vi "Sam_OpenVINO_advanced.vi"() -> ()   [LabVIEW 2018]
doc: "Sam_OpenVINO_Advanced: This example showcases advanced segmentation capabilities using the SAM (Segment Anything Model) integrated with OpenVINO for optimized performance. This implementation enables precise and customizable image segmentation, allowing users to:\n\nSelect Regions of Interest (ROI): Define areas of interest to focus on specific parts of the image for segmentation.\nExclude Regions of Non-Interest: Mark areas to exclude from segmentation, providing flexibility to ignore irrelevant regions.\nCustomizable Segmentation Regions: Choose specific segments within the image for detailed analysis or processing.\nThis advanced segmentation functionality is particularly useful for applications such as medical imaging, industrial inspection, and autonomous systems, where detailed and flexible segmentation is critical. OpenVINO ensures efficient real-time inference, making it suitable for large-scale deployment across diverse hardware platforms."
uses:
  vi.lib/VIRobotics/ModelZoo/Segmentation/Segment_Anything_Utils/sam_mode.ctl
  vi.lib/VIRobotics/opencv_yiku/ctls/ColorConversionCodes.ctl
  vi.lib/VIRobotics/ModelZoo/Segmentation/Segment_Anything_OpenVINO/Segment_Anything_OpenVINO.lvclass
  C:/Program Files/National Instruments/LabVIEW 2018/vi.lib/VIRobotics/ModelZoo/Segmentation/Segment_Anything_Utils/Segment_Anything_Utils.lvclass
  vi.lib/VIRobotics/opencv_yiku/Mat/Mat_8U/Mat_8U.lvclass
  C:/Program Files/National Instruments/LabVIEW 2018/vi.lib/VIRobotics/opencv_yiku/Mat/Mat/Mat.lvclass
  vi.lib/VIRobotics/ModelZoo/Segmentation/Segment_Anything_Utils/set_mode.vi
  vi.lib/VIRobotics/opencv_yiku/Mat/Create_Mat_8U.vi
  vi.lib/VIRobotics/ModelZoo/Segmentation/Segment_Anything_Utils/set_point.vi
  vi.lib/VIRobotics/ModelZoo/Segmentation/Segment_Anything_Utils/set_labels.vi
  vi.lib/VIRobotics/opencv_yiku/Mat/Create_Mat_8UC3_Size.vi
  vi.lib/VIRobotics/opencv_yiku/Mat/Mat/Mat_release.vi
  vi.lib/VIRobotics/opencv_yiku/Mat/Mat/Mat.lvclass
  vi.lib/VIRobotics/opencv_yiku/opencv_yiku.lvlib
  vi.lib/VIRobotics/ModelZoo/Segmentation/Segment_Anything_Utils/Segment_Anything_Utils.lvclass
panel:
  in  "point type":T1(ring)=enum."included"
  in  "decodr_config":cluster{"decoder_model":path, "device":string}={"decoder_model"=path "C:/ProgramData/VIRobotics/ModelZoo/Segmentation/sam/sam-b-dec.onnx", "device"="CPU"}
  in  "encoder_config":cluster{"encoder_model":path, "device":string}={"encoder_model"=path "C:/ProgramData/VIRobotics/ModelZoo/Segmentation/sam/sam-b-enc.onnx", "device"="CPU"}
  in  "img":path=path "C:/ProgramData/VIRobotics/ModelZoo/Segmentation/imgs/plant.jpg"
  out "picture":picture
  out "x-y":dbl
  out "mask":picture
  in  "run":bool
  # "Overview: Demonstrates how to use the VIRobotics openvino toolkit to load the ONNX model of sam for Semantic segmentation annotation\nRequirements: Windows.\nInstructions: \n1.Run the VI.\n2.Specify the image that requires segmentation annotation。\n3.Specify the point type.\n4.Click on the target with the mouse on the picture control\n5.Click run"
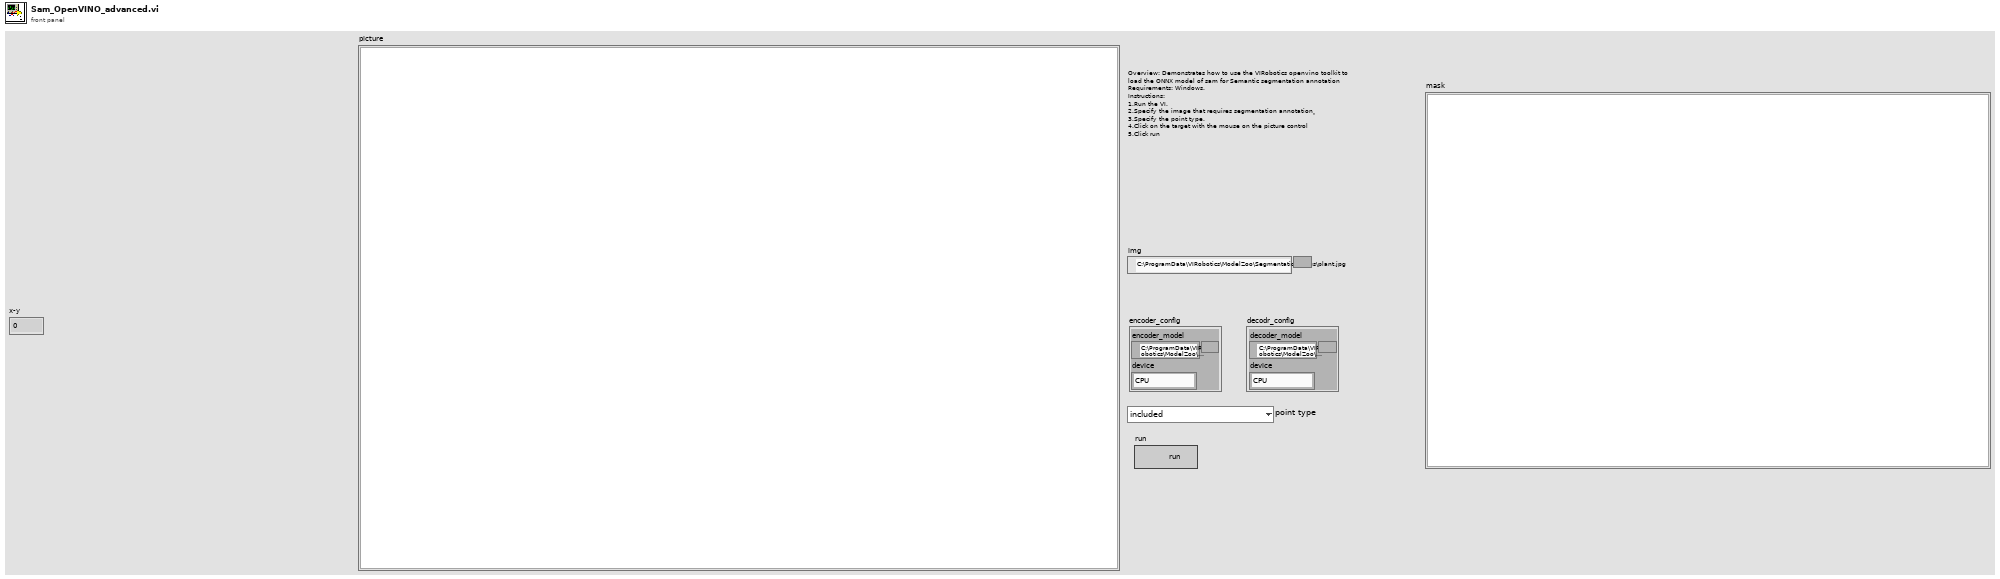
[diagram p1: front panel]
types:
  T1 = enum16{"not included", "included", "top left corner", "bottom right corner"}
  T2 = typedef "Segment_Anything_Utils.lvclass/sam_mode.ctl" = enum16{"points", "box_point", "customize"}
  T3 = typedef "opencv_yiku.lvlib/ColorConversionCodes.ctl" = enum32{"COLOR_BGR2BGRA", "COLOR_BGRA2BGR", "COLOR_BGR2RGBA", "COLOR_RGBA2BGR", "COLOR_BGR2RGB", "COLOR_BGRA2RGBA", "COLOR_BGR2GRAY", "COLOR_RGB2GRAY", "COLOR_GRAY2BGR", "COLOR_GRAY2BGRA", "COLOR_BGRA2GRAY", "COLOR_RGBA2GRAY", "COLOR_BGR2BGR565", "COLOR_RGB2BGR565", "COLOR_BGR5652BGR", "COLOR_BGR5652RGB", "COLOR_BGRA2BGR565", "COLOR_RGBA2BGR565", "COLOR_BGR5652BGRA", "COLOR_BGR5652RGBA", "COLOR_GRAY2BGR565", "COLOR_BGR5652GRAY", "COLOR_BGR2BGR555", "COLOR_RGB2BGR555", "COLOR_BGR5552BGR", "COLOR_BGR5552RGB", "COLOR_BGRA2BGR555", "COLOR_RGBA2BGR555", "COLOR_BGR5552BGRA", "COLOR_BGR5552RGBA", "COLOR_GRAY2BGR555", "COLOR_BGR5552GRAY", "COLOR_BGR2XYZ", "COLOR_RGB2XYZ", "COLOR_XYZ2BGR", "COLOR_XYZ2RGB", "COLOR_BGR2YCrCb", "COLOR_RGB2YCrCb", "COLOR_YCrCb2BGR", "COLOR_YCrCb2RGB", "COLOR_BGR2HSV", "COLOR_RGB2HSV", "42", "43", "COLOR_BGR2Lab", "COLOR_RGB2Lab"}
  T4 = typedef "LVBoundsTypeDef.ctl" = cluster{"Width":u32, "Height":u32}
  T5 = typedef "LVMouseTypeDef.ctl" = cluster{"Mouse Position":cluster{"X":i32, "Y":i32}, "Mouse Modifiers":cluster{"Button Down":bool, "Shift Mod":bool, "Menu Mod":bool, "Option Mod":bool}}
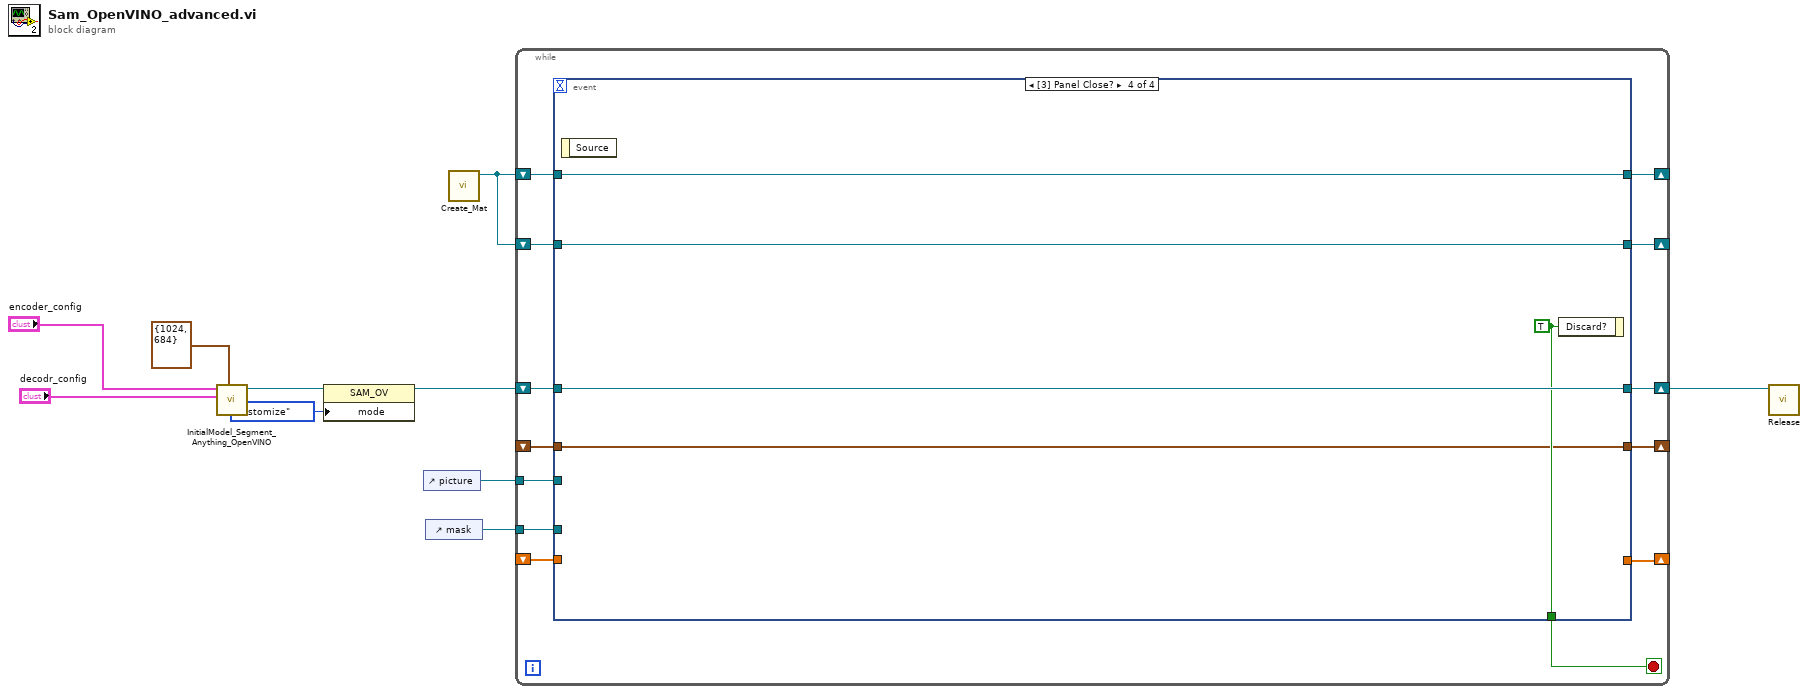
[diagram p0: block diagram]
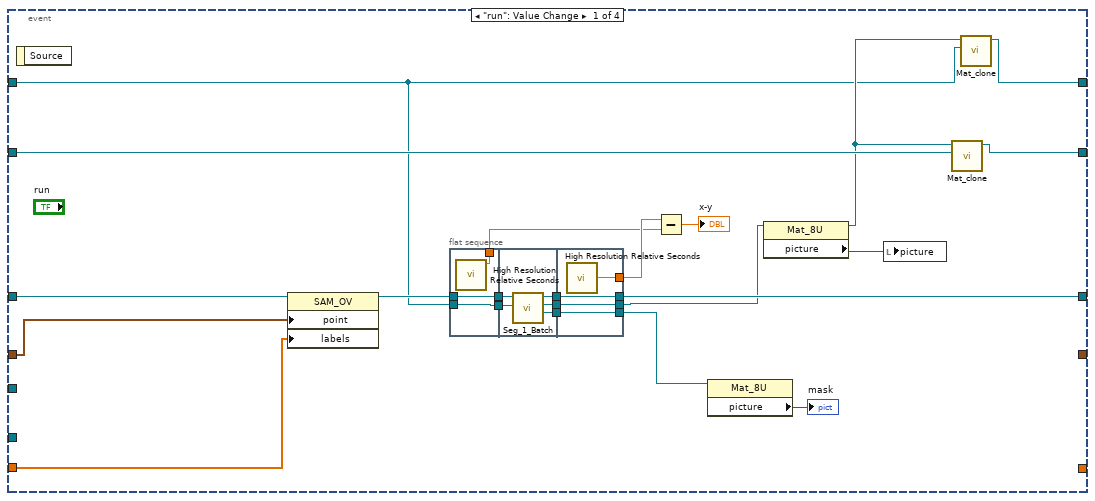
[diagram p2: hidden frame]
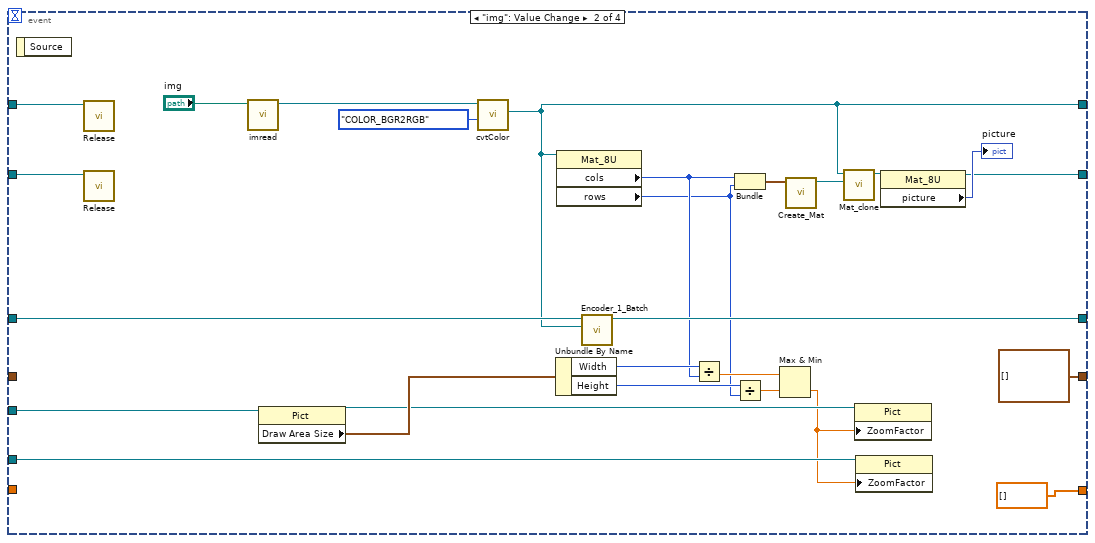
[diagram p3: hidden frame]
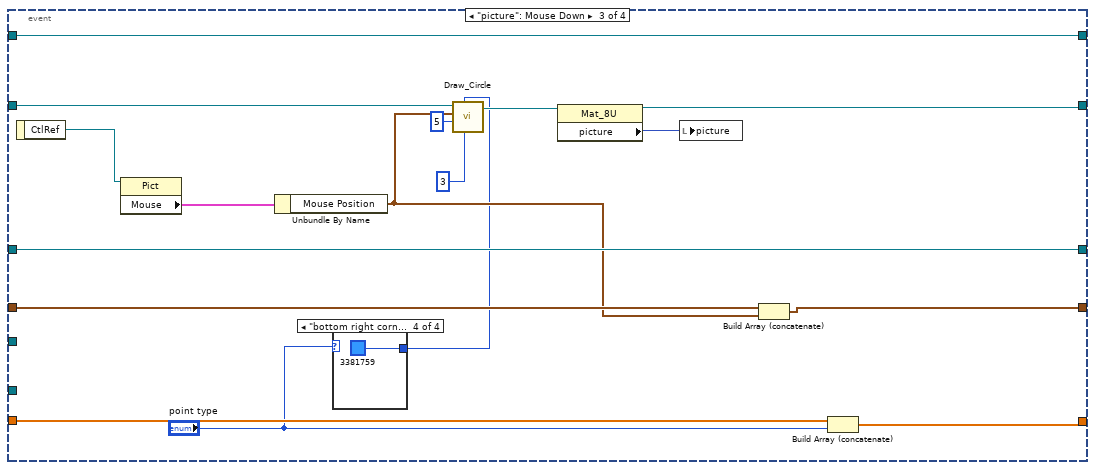
[diagram p4: hidden frame]
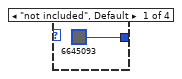
[diagram p5: hidden frame]
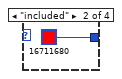
[diagram p6: hidden frame]
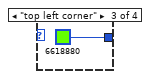
[diagram p7: hidden frame]
diagram:
  n1 = call "InitialModel_Segment_Anything_OpenVINO.vi"("inputSize"=cluster{"x":i32, "y":i32} {"x"=1024, "y"=684} ("Size"), "decodr_config"="decodr_config", "encoder_config"="encoder_config") -> ("SAM_OV out"=w3:refnum<class "Segment_Anything_OpenVINO.lvclass">)  [unwired: 7 in, 1 out]
  n2 = property class="SAM_OV"(reference=w3, "mode"=sam_mode."customize") -> (reference out=w2:refnum<class "Segment_Anything_OpenVINO.lvclass">)  [unwired: 1 in, 1 out]
  n3 = control-ref of="picture"() -> (w9:refnum<vi>)
  n4 = control-ref of="mask"() -> (w8:refnum<vi>)
  n5 = call-poly "Create_Mat.vi"() -> ("Mat_8U_out"=w7:refnum<class "Mat_8U.lvclass">)  [unwired: 10 in, 1 out]
  n6 = while {
    shift-right: [w22] -> w10
    shift-left: w2 -> [w23]
    tunnel: w9 -> [w20]
    shift-right: [w19] -> _
    shift-left: w7 -> [w18]
    tunnel: w8 -> [w17]
    shift-right: [w16] -> _
    shift-left: _ -> [w15]
    shift-right: [w14] -> _
    shift-left: w7 -> [w13]
    shift-right: [w12] -> _
    shift-left: _ -> [w11]
    stop <- w21 stop-if-true
    n7 = event shown="[3] Panel Close?" {
      selector: _ -> [_ _ _ _]
      dyn-events: _ -> [_ _ _ _]
      timeout: _ -> [_ _ _ _]
      tunnel: w23 -> [w36 w82 w89 w109]
      tunnel: [w34 w81 w89 w109] -> w22
      tunnel: [_ _ _ w108] -> w21
      tunnel: w20 -> [_ w78 _ _]
      tunnel: [w26 w65 w99 w106] -> w19
      tunnel: w18 -> [w27 w71 w99 w106]
      tunnel: w17 -> [_ w60 _ _]
      tunnel: [_ cluster{"x":sgl, "y":sgl}[] [] w92 w107] -> w16
      tunnel: w15 -> [w25 _ w93 w107]
      tunnel: [w29 w62 w90 w105] -> w14
      tunnel: w13 -> [w30 w61 w91 w105]
      tunnel: [_ sgl[] [] w86 _] -> w12
      tunnel: w11 -> [w24 _ w87 _]
      event "run": Value Change {
        n8 = event-data() -> ()  [unwired: 1 in, 1 out]
        n9 = property class="SAM_OV"(reference=w36, "point"=w25, "labels"=w24) -> (reference out=w35:refnum<class "Segment_Anything_OpenVINO.lvclass">)  [unwired: 1 in, 1 out]
        n10 = flat-sequence {
          tunnel: w35 -> [w48]
          tunnel: [w48] -> w45
          tunnel: [w47] -> w40
          tunnel: w27 -> [w46]
          tunnel: [w46] -> w33
          tunnel: w45 -> [w53]
          tunnel: [w52] -> w44
          tunnel: [w51] -> w43
          tunnel: [w50] -> w42
          tunnel: w33 -> [w49]
          tunnel: [w56] -> w32
          tunnel: [w57] -> w34
          tunnel: w44 -> [w57]
          tunnel: w43 -> [w56]
          tunnel: [w55] -> w41
          tunnel: [w54] -> w38
          tunnel: w42 -> [w54]
          frame #0 {
            n11 = call <vilib>:"High Resolution Relative Seconds.vi"() -> ("relative seconds"=w47:dbl)
          }
          frame #1 {
            n12 = call-dynamic "Seg_1_Batch.vi"("img"=w49, "Segment_Anything_OpenVINO in"=w53) -> ("mask"=w50:refnum<class "Mat_8U.lvclass">, "img out"=w51:refnum<class "Mat_8U.lvclass">, "Segment_Anything_OpenVINO out"=w52:refnum<class "Segment_Anything_OpenVINO.lvclass">)  [unwired: 6 in, 1 out]
          }
          frame #2 {
            n13 = call <vilib>:"High Resolution Relative Seconds.vi"() -> ("relative seconds"=w55:dbl)
          }
        }
        n14 = Subtract(x=w41, y=w40) -> (x-y=→"x-y":dbl)
        n15 = property class="Mat_8U"(reference=w38) -> ("picture"=→"mask":picture)  [unwired: 1 in, 2 out]
        n16 = property class="Mat_8U"(reference=w32) -> (reference out=w28:refnum<class "Mat_8U.lvclass">, "picture"=w31:picture)  [unwired: 1 in, 1 out]
        n17 = local write "picture"(w31) -> ()
        n18 = call "Mat_clone.vi"("dst"=w30, "Mat in"=w28) -> ("dst 2"=w29:refnum<class "Mat_8U.lvclass">)  [unwired: 8 in, 1 out]
        n19 = call "Mat_clone.vi"("dst"=w27, "Mat in"=w28) -> ("dst 2"=w26:refnum<class "Mat_8U.lvclass">)  [unwired: 8 in, 1 out]
      }
      event "img": Value Change {
        n20 = event-data() -> ()  [unwired: 1 in, 1 out]
        n21 = call-poly "Release.vi"("Mat in"=w71) -> ()  [unwired: 10 in, 1 out]
        n22 = call-poly "Release.vi"("Mat in"=w61) -> ()  [unwired: 10 in, 1 out]
        n23 = call "imread.vi"("path"="img") -> ("Mat out"=w80:refnum<class "Mat_8U.lvclass">)  [unwired: 9 in, 1 out]
        n24 = property class="Pict"(reference=w78) -> (reference out=w72:refnum<vi>, "Draw Area Size"=w77:T4)  [unwired: 1 in, 1 out]
        n25 = call "cvtColor.vi"("dstCn"=ColorConversionCodes."COLOR_BGR2RGB", "src"=w80) -> ("dst out"=w65:refnum<class "Mat_8U.lvclass">)  [unwired: 7 in, 2 out]
        n26 = Unbundle By Name(w77) -> ("Width"=w76:u32, "Height"=w75:u32)
        n27 = property class="Mat_8U"(reference=w65) -> ("cols"=w69:i32, "rows"=w68:i32)  [unwired: 1 in, 2 out]
        n28 = call-dynamic "Encoder_1_Batch.vi"("image"=w65, "SAM_OV in"=w82) -> ("SAM_OV out"=w81:refnum<class "Segment_Anything_OpenVINO.lvclass">)  [unwired: 8 in, 1 out]
        n29 = Divide(x=w76, y=w69) -> (x/y=w73:dbl)
        n30 = Bundle("cols"=w69, "rows"=w68) -> (w67:cluster{"cols":i32, "rows":i32})  [unwired: 1 in]
        n31 = Divide(x=w75, y=w68) -> (x/y=w74:dbl)
        n32 = Max & Min(x=w73, y=w74) -> (min(x,y)=w59:dbl)  [unwired: 1 out]
        n33 = call-poly "Create_Mat.vi"("Size"=w67) -> ("Mat_8U_out"=w66:refnum<class "Mat_8U.lvclass">)  [unwired: 9 in, 1 out]
        n34 = call "Mat_clone.vi"("dst"=w66, "Mat in"=w65) -> ("dst 2"=w64:refnum<class "Mat_8U.lvclass">)  [unwired: 8 in, 1 out]
        n35 = property class="Pict"(reference=w72, "ZoomFactor"=w59) -> ()  [unwired: 1 in, 2 out]
        n36 = property class="Pict"(reference=w60, "ZoomFactor"=w59) -> ()  [unwired: 1 in, 2 out]
        n37 = property class="Mat_8U"(reference=w64) -> (reference out=w62:refnum<class "Mat_8U.lvclass">, "picture"=→"picture":picture)  [unwired: 1 in, 1 out]
      }
      event "picture": Mouse Down {
        n38 = event-data() -> ("CtlRef"=w100:refnum<vi>)  [unwired: 1 in]
        n39 = property class="Pict"(reference=w100) -> ("Mouse"=w98:T5)  [unwired: 1 in, 2 out]
        n40 = Unbundle By Name(w98) -> ("Mouse Position"=w88:cluster{"X":i32, "Y":i32})
        n41 = case shown="\"bottom right corner\"" "point type" {
          tunnel: [u32 6645093 ("color(black)") u32 16711680 ("color(black)") u32 6618880 ("color(black)") u32 3381759 ("color(black)")] -> w85
          frame "not included", Default {
          }
          frame "included" {
          }
          frame "top left corner" {
          }
          frame "bottom right corner" {
          }
        }
        n42 = call "Draw_Circle.vi"("thickness"=3, "color"=w85, "radius"=5, "center"=w88, "Mat"=w91) -> ("Mat out"=w95:refnum<class "Mat_8U.lvclass">)  [unwired: 5 in, 1 out]
        n43 = property class="Mat_8U"(reference=w95) -> (reference out=w90:refnum<class "Mat_8U.lvclass">, "picture"=w94:picture)  [unwired: 1 in, 1 out]
        n44 = local write "picture"(w94) -> ()
        n45 = Build Array (concatenate)(w93, w88) -> (w92:cluster{"x":sgl, "y":sgl}[])
        n46 = Build Array (concatenate)(w87, "point type") -> (w86:sgl[])
      }
      event Panel Close? {
        w108 = TRUE ("Discard?")
        n47 = event-data() -> ()  [unwired: 1 in, 1 out]
        n48 = event-data("Discard?"=w108) -> ()  [unwired: 1 in, 1 out]
      }
    }
  }
  n49 = call-dynamic "Release.vi"("Segment_Anything_OpenVINO in"=w10) -> ()  [unwired: 9 in, 2 out]
